vi "Acquire Class Details.vi"(8 "error in":errorcluster, 11 "Class Path":path) -> (0 "error out":errorcluster, 1 "Member VI info":T2[](array[typedef]), 2 "Hierarchy Array":T1[](array[typedef]), 3 "Class Info":T1, 5 "Is Interface":bool)   [LabVIEW 2019, in "ClassLoader.lvlib"]
doc: "Obtain class data using VI server."
uses:
  ClassLoader.lvlib
  Ctl/Ctl_Class Info.ctl
  <vilib>/Utility/Data Type/Member VI Info.ctl
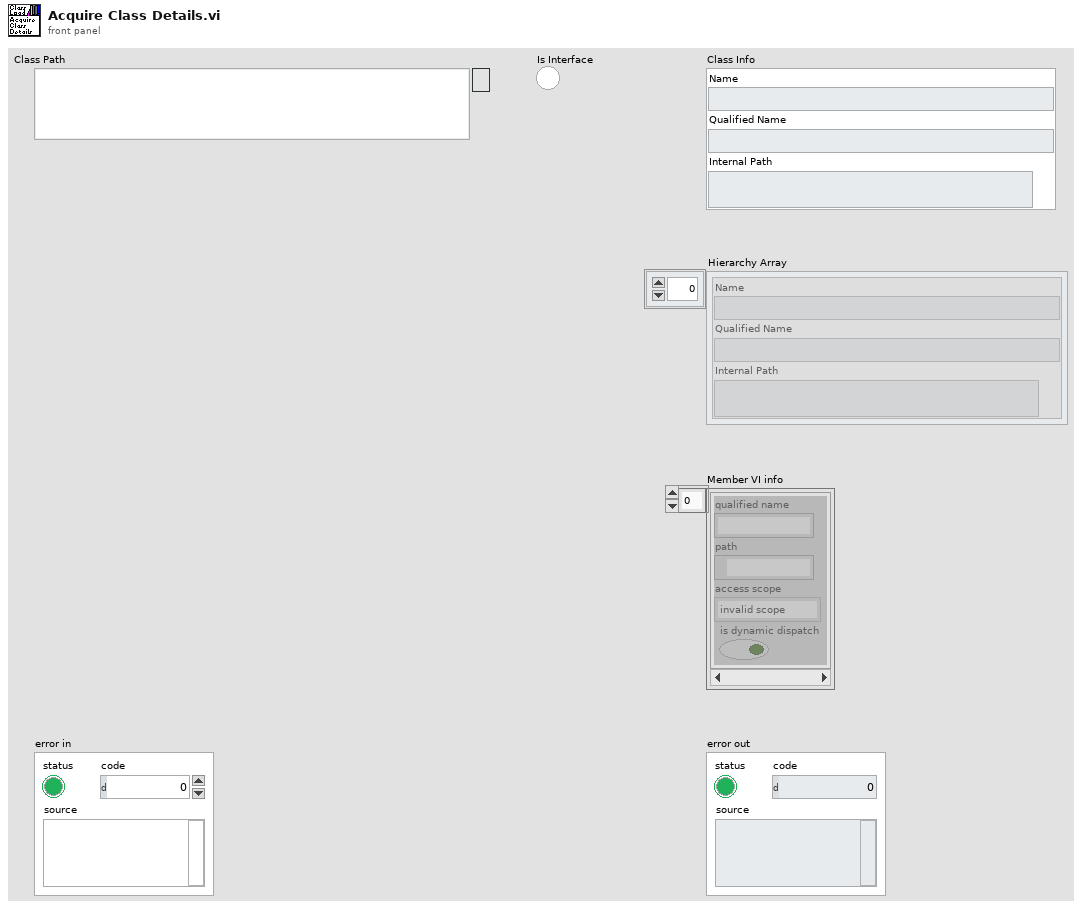
[diagram p1: front panel]
types:
  T1 = typedef "ClassLoader.lvlib/Ctl_Class Info.ctl" = cluster{"Name":string, "Qualified Name":string, "Internal Path":string}
  T2 = typedef "Member VI Info.ctl" = cluster{"qualified name":string, "path":path, "access scope":enum32{"invalid scope", "public", "private", "protected", "community"}, "is dynamic dispatch":bool}
  T3 = cluster{"Static Member VIs":refnum<vi>[], "is dynamic dispatch":bool}
  T4 = cluster{"Dynamic Member VIs":refnum<vi>[], "is dynamic dispatch":bool}
  T5 = cluster{"Dynamic Member VIs":refnum<vi>[], "is dynamic dispatch":bool}[]
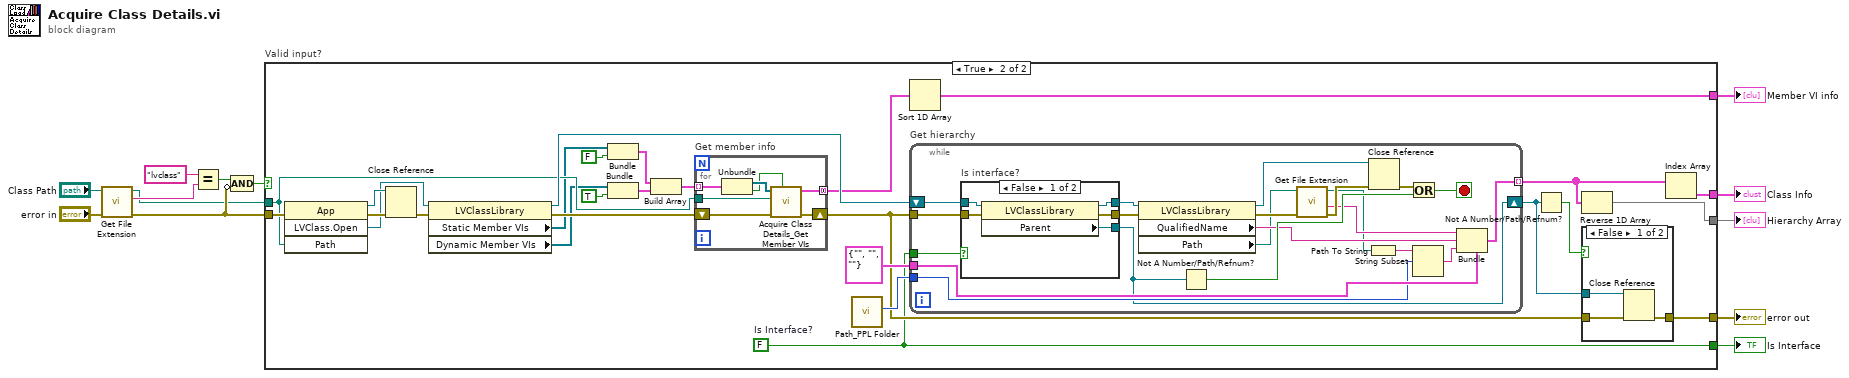
[diagram p0: block diagram]
diagram:
  n1 = call <vilib>:"Get File Extension.vi"("error in (no error)"="error in", "file"="Class Path") -> ("error out"=w7:errorcluster, "lowercase file extension"=w13:string, "dup file"=w6:path)  [unwired: 5 in, 2 out]
  n2 = Equal?(x="lvclass", y=w13) -> (x = y?=w11:bool)
  n3 = Compound Arithmetic op=AND(w11, invert w7) -> (w9:bool)
  n4 = case "Valid input?" shown="True" w9 {
    tunnel: [w14 w38] -> w8
    tunnel: w7 -> [w14 w39]
    tunnel: w6 -> [_ w25]
    tunnel: [_ w37] -> w5
    tunnel: [_ w29] -> w4
    tunnel: [_ w15] -> w3
    tunnel: [_ w27] -> w2
    frame False {
    }
    frame True {
      w15 = FALSE  # Is Interface?
      n5 = invoke class="App" method="LVClass.Open"(error in=w39, "Path"=w25) -> (reference out=w40:refnum<vi>, error out=w41:errorcluster, "LVClass.Open"=w34:refnum<vi>)  [unwired: 2 in, 1 out]
      n6 = Close Reference(reference=w40, error in (no error)=w41) -> (error out=w32:errorcluster)
      n7 = property class="LVClassLibrary"(reference=w34, error in=w32) -> (reference out=w33:refnum<vi>, error out=w31:errorcluster, "Static Member VIs"=w23:refnum<vi>[], "Dynamic Member VIs"=w20:refnum<vi>[])
      n8 = Bundle("Static Member VIs"=w23, "is dynamic dispatch"=FALSE) -> (w19:T3)  [unwired: 1 in]
      n9 = Bundle("Dynamic Member VIs"=w20, "is dynamic dispatch"=TRUE) -> (w18:T4)  [unwired: 1 in]
      n10 = Build Array(w19, w18) -> (w17:T5)
      n11 = for "Get member info" {
        tunnel: [w46] -> w30 mode=concatenating
        tunnel: w25 -> [w45]
        shift-right: [w47] -> w16
        shift-left: w31 -> [w48]
        tunnel: w17 -> [w44] mode=indexing
        n12 = Unbundle(w44) -> ("Dynamic Member VIs"=w43:refnum<vi>[], "is dynamic dispatch"=w42:bool)
        n13 = call "Acquire Class Details_Get Member VIs.vi"("Dynamic dispatch?"=w42, "error in (no error)"=w48, "Class Path"=w45, "Member VIs (auto closed)"=w43) -> ("error out"=w47:errorcluster, "Member Array"=w46:T2[])  [unwired: 6 in]
      }
      n14 = call "Path_PPL Folder.vi"() -> ("Path Length"=w24:i32)  [unwired: 10 in, 1 out]
      n15 = Sort 1D Array(array=w30) -> (sorted array=w29:T2[])
      n16 = while "Get hierarchy" {
        shift-right: [w56] -> w36
        shift-left: w33 -> [w58]
        tunnel: [w72] -> w28 mode=indexing
        tunnel: w16 -> [w54]
        tunnel: T1 {"Name"="", "Qualified Name"="", "Internal Path"=""} ("Class Info") -> [w63]
        tunnel: w24 -> [w61]
        tunnel: w15 -> [w53]
        stop <- w70 stop-if-true
        n17 = case "Is interface?" shown="False" w53 {
          tunnel: w58 -> [w78 w80]
          tunnel: [w77 w80] -> w57
          tunnel: [w76 _] -> w56
          tunnel: [w75 w79] -> w55
          tunnel: w54 -> [w74 w79]
          frame False {
            n18 = property class="LVClassLibrary"(reference=w78, error in=w74) -> (reference out=w77:refnum<vi>, error out=w75:errorcluster, "Parent"=w76:refnum<vi>)
          }
          frame True {
          }
        }
        n19 = property class="LVClassLibrary"(reference=w57, error in=w55) -> (reference out=w67:refnum<vi>, error out=w66:errorcluster, "QualifiedName"=w65:string, "Path"=w64:path)
        n20 = Not A Number/Path/Refnum?(number/path/refnum=w56) -> (NaN/Path/Refnum?=w73:bool)
        n21 = call <vilib>:"Get File Extension.vi"("error in (no error)"=w66, "file"=w64) -> ("error out"=w69:errorcluster, "filename without extension"=w68:string, "dup file"=w60:path)  [unwired: 5 in, 2 out]
        n22 = Path To String(path=w60) -> (string=w62:string)
        n23 = Close Reference(reference=w67, error in (no error)=w69) -> (error out=w71:errorcluster)
        n24 = Or(x=w71, y=w73) -> (x .or. y?=w70:bool)
        n25 = String Subset(string=w62, offset (0)=w61) -> (substring=w59:string)  [unwired: 1 in]
        n26 = Bundle(cluster=w63, "Name"=w68, "Qualified Name"=w65, "Internal Path"=w59) -> (w72:T1)
      }
      n27 = Not A Number/Path/Refnum?(number/path/refnum=w36) -> (NaN/Path/Refnum?=w35:bool)
      n28 = Reverse 1D Array(array=w28) -> (reversed array=w37:T1[])
      n29 = case shown="False" w35 {
        tunnel: w16 -> [w51 w52]
        tunnel: [w50 w52] -> w38
        tunnel: w36 -> [w49 _]
        frame False {
          n30 = Close Reference(reference=w49, error in (no error)=w51) -> (error out=w50:errorcluster)
        }
        frame True {
        }
      }
      n31 = Index Array(array=w28) -> (element=w27:T1)  [unwired: 1 in]
    }
  }
  "error out" <- w8
  "Member VI info" <- w4
  "Hierarchy Array" <- w5
  "Is Interface" <- w3
  "Class Info" <- w2
